vi "Trajectory_AlmostEquals.vi"(6 "Tolerance":dbl=1e-05 format="%#_13g", 9 "other TRAJECTORY":T1 {"States"."POSE"."ROTATION"."SIN" format="%13.4f"; "States"."POSE"."ROTATION"."COS" format="%13.4f"; "States"."POSE"."ROTATION"."VALUE" format="%13.4f"; "States"."POSE"."TRANSLATION"."Y" format="%14.3f"; "States"."POSE"."TRANSLATION"."X" format="%14.3f"; "TotalTImeSecs" format="%20.3f"}, 11 "TRAJECTORY":T1 {"States"."POSE"."ROTATION"."SIN" format="%13.4f"; "States"."POSE"."ROTATION"."COS" format="%13.4f"; "States"."POSE"."ROTATION"."VALUE" format="%13.4f"; "States"."POSE"."TRANSLATION"."Y" format="%14.3f"; "States"."POSE"."TRANSLATION"."X" format="%14.3f"; "TotalTImeSecs" format="%20.3f"}) -> (3 "Equals":bool)   [LabVIEW 2019]
doc: "Determines if two trajectories are equal.\n\nParameters:\n - Trajectory - Trajectory data structure\n - Other Trajectory - Trajectory data structure\n\nReturns:\n - Equals - boolean indicating if the two trajectories are equal."
uses:
  <vilib>/Rock Robotics/WPI/ThirdParty/JAS_Junk/TrajLib/TRAJECTORY.ctl
  <vilib>/Rock Robotics/WPI/ThirdParty/JAS_Junk/TrajLib/TRAJ_STATE.ctl
  <vilib>/Rock Robotics/WPI/ThirdParty/JAS_Junk/TrajLib/POSE2D.ctl
  <vilib>/Rock Robotics/WPI/ThirdParty/JAS_Junk/TrajLib/TRANSLATION2D.ctl
  <vilib>/Rock Robotics/WPI/ThirdParty/JAS_Junk/TrajLib/ROTATION2D.ctl
  Pose_AlmostEquals.vi
  Translation_AlmostEquals.vi
  Rotation_AlmostEquals.vi
  <vilib>/Rock Robotics/WPI/ThirdParty/JAS_Junk/TrajLib/Util_CalcDist.vi
  <vilib>/Rock Robotics/WPI/ThirdParty/JAS_Junk/TrajLib/Trajectory_Library.lvlib
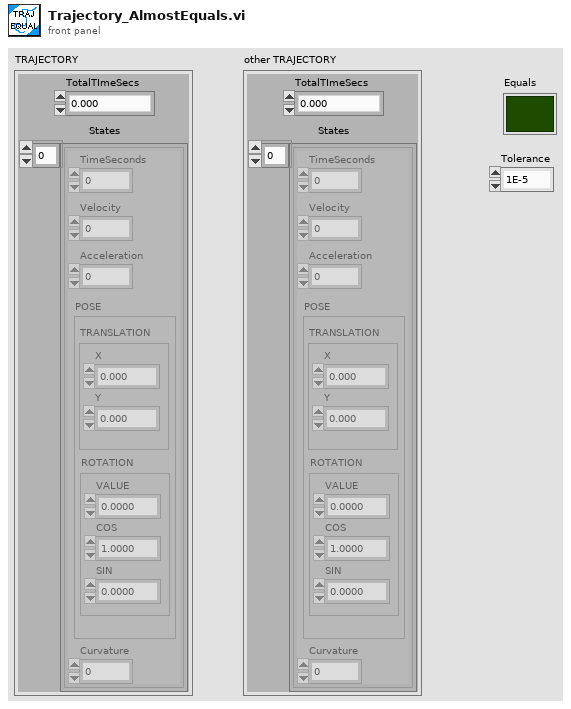
[diagram p1: front panel]
types:
  T1 = typedef "Trajectory_Library.lvlib/TRAJECTORY.ctl" = cluster{"TotalTImeSecs":dbl, "States":T2[]}
  T2 = typedef "Trajectory_Library.lvlib/TRAJ_STATE.ctl" = cluster{"TimeSeconds":dbl, "Velocity":dbl, "Acceleration":dbl, "POSE":T3, "Curvature":dbl}
  T3 = typedef "Trajectory_Library.lvlib/POSE2D.ctl" = cluster{"TRANSLATION":T4, "ROTATION":T5}
  T4 = typedef "Trajectory_Library.lvlib/TRANSLATION2D.ctl" = cluster{"X":dbl, "Y":dbl}
  T5 = typedef "Trajectory_Library.lvlib/ROTATION2D.ctl" = cluster{"VALUE":dbl, "COS":dbl, "SIN":dbl}
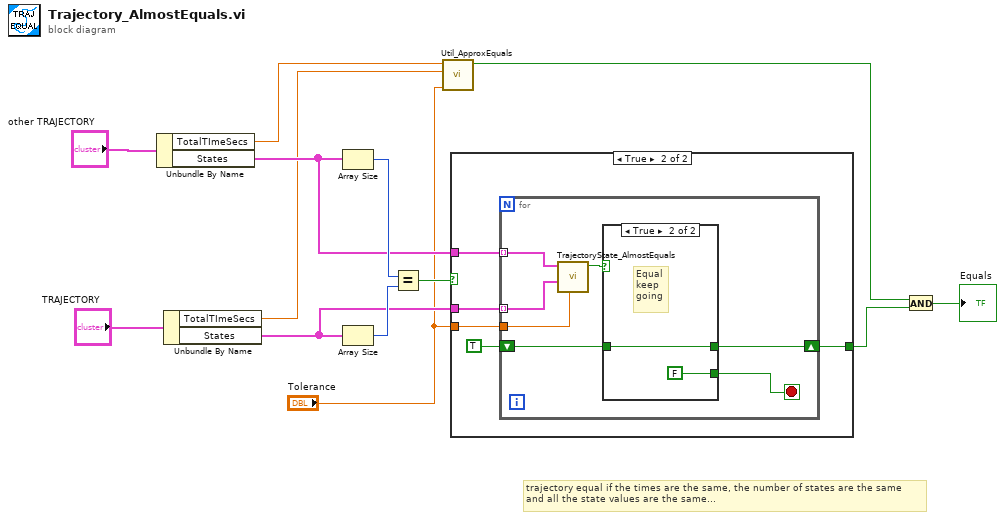
[diagram p0: block diagram]
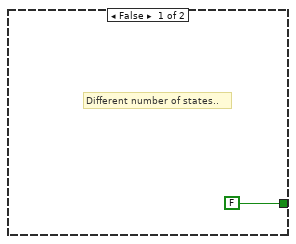
[diagram p2: hidden frame]
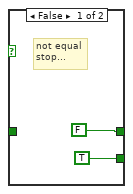
[diagram p3: hidden frame]
diagram:
  # "trajectory equal if the times are the same, the number of states are the same\nand all the state values are the same..."
  n1 = Unbundle By Name("other TRAJECTORY") -> ("TotalTImeSecs"=w4:dbl, "States"=w7:T2[])
  n2 = Unbundle By Name("TRAJECTORY") -> ("TotalTImeSecs"=w3:dbl, "States"=w8:T2[])
  n3 = Array Size(array=w7) -> (size(s)=w11:i32)
  n4 = Array Size(array=w8) -> (size(s)=w10:i32)
  n5 = Equal?(x=w11, y=w10) -> (x = y?=w9:bool)
  n6 = call <vilib>:"Util_ApproxEquals.vi"("Tolerance"="Tolerance", "Value 2"=w3, "Value 1"=w4) -> ("ApproxEquals"=w1:bool)  [unwired: 8 in]
  n7 = case shown="True" w9 {
    tunnel: [FALSE w18] -> w6
    tunnel: w8 -> [_ w17]
    tunnel: w7 -> [_ w16]
    tunnel: "Tolerance" -> [_ w15]
    frame False {
      # "Different number of states.."
    }
    frame True {
      n8 = for {
        shift-right: [w22] -> w18
        shift-left: TRUE -> [w23]
        tunnel: w17 -> [w25] mode=indexing
        tunnel: w16 -> [w26] mode=indexing
        tunnel: w15 -> [w20]
        stop <- w21 stop-if-true
        n9 = call "TrajectoryState_AlmostEquals.vi"("Tolerance"=w20, "Other TRAJ_STATE"=w25, "TRAJ_STATE"=w26) -> ("Equals"=w24:bool)  [unwired: 8 in]
        n10 = case shown="True" w24 {
          tunnel: w23 -> [_ w30]
          tunnel: [FALSE w30] -> w22
          tunnel: [TRUE FALSE] -> w21
          frame False {
            # "not equal\nstop..."
          }
          frame True {
            # "Equal\nkeep\ngoing"
          }
        }
      }
    }
  }
  n11 = And(x=w1, y=w6) -> (x .and. y?=→"Equals":bool)
